vi "Stop SSH Module.vi"(6 "Wait for Module to stop? (F)":bool, 7 "Connection Name":string, 8 "error in (no error)":errorcluster, 9 "Origin":string, 10 "Module ID":i32=-1) -> (0 "error out":errorcluster)   [LabVIEW 2017]
doc: "Use either Connection Name or Module ID to specify a module to stop. If nothing is selected, default value of Module ID is -1, which will stop all SSH client modules."
uses:
  Libraries/SSH/SSH.lvlib
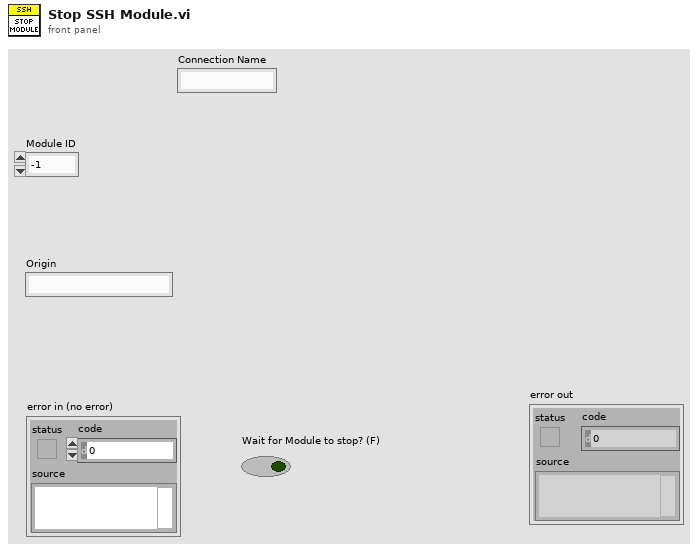
[diagram p1: front panel]
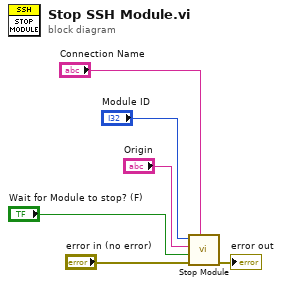
[diagram p0: block diagram]
diagram:
  n1 = call "Stop Module.vi"("Connection Name"="Connection Name", "error in (no error)"="error in (no error)", "Wait for Module to stop? (F)"="Wait for Module to stop? (F)", "Origin"="Origin", "Module ID"="Module ID") -> ("error out"=→"error out":errorcluster)  [unwired: 6 in]
